vi "Serial_Get_Ref.vi"(3 "error in (no error)":errorcluster) -> (0 "error out":errorcluster, 2 "Serial Ref":T2)   [LabVIEW 2009, in "Serial.lvlib"]
doc: "Provides a Serial reference to use."
uses:
  Serial.lvlib
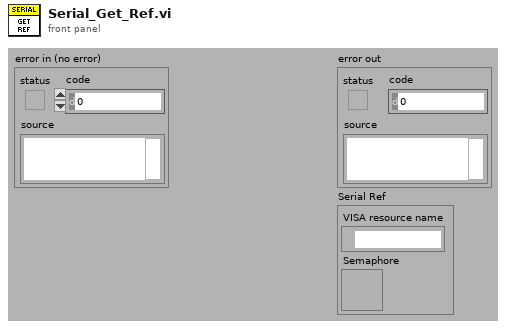
[diagram p1: front panel]
types:
  T1 = typedef "Semaphore RefNum" = refnum<k1>
  T2 = cluster{"VISA resource name":refnum<visa-resource-name>, "Semaphore":T1}
  T3 = cluster{"VISA resource name":refnum<visa-resource-name>, "Semaphore":refnum<k1>}
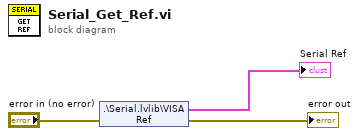
[diagram p0: block diagram]
diagram:
  n1 = shared-variable ".\\Serial.lvlib\\VISA Ref"(error in="error in (no error)") -> (→"Serial Ref":T3, error out=→"error out":errorcluster)
